vi "Demo.vi"() -> ()   [LabVIEW 2013, in "LV Process library.lvlib"]
doc: "Demonstartion of basic use of LV Process library. Starts process 'cmd', writes a buffer and reads output.\n\n---\nLV Process works only with lv_proc.dll library, which is part of vipm package or should be delivered together with packed library. Placement of this dll is selected in terminal of Create Process.vi."
uses:
  LV Process library.lvlib
panel:
  out "lv_proc.dll version":string
  in  "write buffer - command to quit process:":string="exit\n"
  out "debug data":T1(array[cluster])
  in  "read buffer byte count:":i32=1024
  in  "wait for exit timeout [ms]:":i32=10
  in  "write buffer:":string="date /T\n"
  out "read buffer:":string
  out "bytes written:":i32
  out "exit code:":i32
  out "error out":errorcluster
  in  "command:":string="cmd"
  in  "working directory:":string="c:\\"
  # "LV Process demo\n\nWhat demo does?"
  # "1,\nStarts windows command\nline by command 'cmd' in\nworking directory 'c:\\'."
  # "2,\nWrites command\n'date /T' to stdin."
  # "4,\nWaits 200 ms,\nreads output of stdout."
  # "5,\nWrites command 'exit' to end \nthe process,\nwaits 10 ms for process exit,\nclean up pipe handle."
  # "6,\nAs debugging was enabled in the pipe handle cluster,\nall writes to stdin and readings of stdout are stored in the pipe handle cluster."
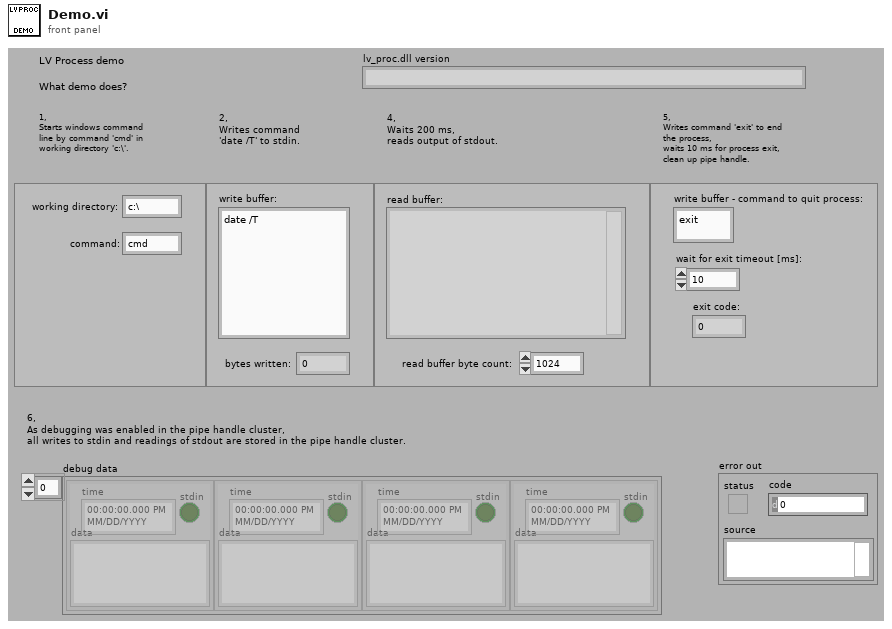
[diagram p1: front panel]
types:
  T1 = cluster{"time":timestamp, "stdin":bool, "data":string}[]
  T2 = typedef "LV Process library.lvlib/Pipe Handle.ctl" = cluster{"lv_proc.dll file path":path, "process instance handle":u32[], "debug mode":bool, "debug data":cluster{"time":timestamp, "stdin":bool, "data":string}[]}
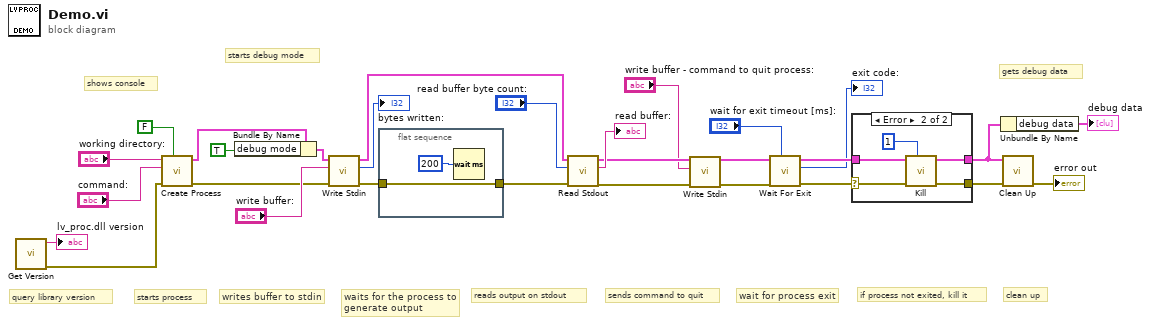
[diagram p0: block diagram]
diagram:
  # "query library version"
  # "waits for the process to\ngenerate output"
  # "shows console"
  # "sends command to quit"
  # "gets debug data"
  # "starts debug mode"
  # "clean up"
  # "if process not exited, kill it"
  # "wait for process exit"
  # "reads output on stdout"
  # "writes buffer to stdin"
  # "starts process"
  n1 = call "Get Version.vi"() -> ("error out"=w1:errorcluster, "version"=→"lv_proc.dll version":string)  [unwired: 10 in]
  n2 = call "Create Process.vi"("hide window (T)"=FALSE, "error in"=w1, "command"="command:", "working directory"="working directory:") -> ("error out"=w16:errorcluster, "pipe out"=w13:T2)  [unwired: 6 in]
  n3 = Bundle By Name(cluster=w13, "debug mode"=TRUE) -> (w11:T2)
  n4 = call "Write Stdin.vi"("error in"=w16, "write buffer"="write buffer:", "pipe in"=w11) -> ("error out"=w14:errorcluster, "return count"=→"bytes written:":i32, "pipe out"=w24:T2)  [unwired: 6 in]
  n5 = flat-sequence {
    tunnel: [w30] -> w15
    tunnel: w14 -> [w30]
    frame #0 {
      n6 = Wait (ms)(milliseconds to wait=u32 200) -> ()  [unwired: 1 out]
    }
  }
  n7 = call "Read Stdout.vi"("error in"=w15, "byte count"="read buffer byte count:", "pipe in"=w24) -> ("error out"=w6:errorcluster, "read buffer"=→"read buffer:":string, "pipe out"=w7:T2)  [unwired: 3 in, 3 out]
  n8 = call "Write Stdin.vi"("error in"=w6, "write buffer"="write buffer - command to quit process:", "pipe in"=w7) -> ("error out"=w5:errorcluster, "pipe out"=w4:T2)  [unwired: 6 in, 1 out]
  n9 = call "Wait For Exit.vi"("timeout [ms] (1)"="wait for exit timeout [ms]:", "error in"=w5, "pipe in"=w4) -> ("error out"=w22:errorcluster, "exit code"=→"exit code:":i32, "pipe out"=w26:T2)  [unwired: 6 in]
  n10 = case shown="Error" w22 {
    selector: w22 -> [w32 w34]
    tunnel: w26 -> [w33 w38]
    tunnel: [w32 w35] -> w21
    tunnel: [w33 w36] -> w10
    frame No Error {
    }
    frame Error {
      n11 = call "Kill.vi"("timeout [ms]"=1, "error in"=w34, "pipe in"=w38) -> ("error out"=w35:errorcluster, "pipe out"=w36:T2)  [unwired: 7 in]
    }
  }
  n12 = Unbundle By Name(w10) -> ("debug data"=→"debug data":T1)
  n13 = call "Clean Up.vi"("error in"=w21, "pipe in"=w10) -> ("error out"=→"error out":errorcluster)  [unwired: 9 in]
